vi "DataLogger_WriteData.vi"(8 "error in (no error)":errorcluster, 10 "New line":string, 11 "Data Logger in":refnum<class "Data Logger.lvclass">) -> (0 "error out":errorcluster, 3 "Data Logger out":refnum<class "Data Logger.lvclass">)   [LabVIEW 2015, in "Data Logger.lvclass"]
uses:
  Data Logger.lvclass
  Data Logger.lvclass/Data Logger.ctl
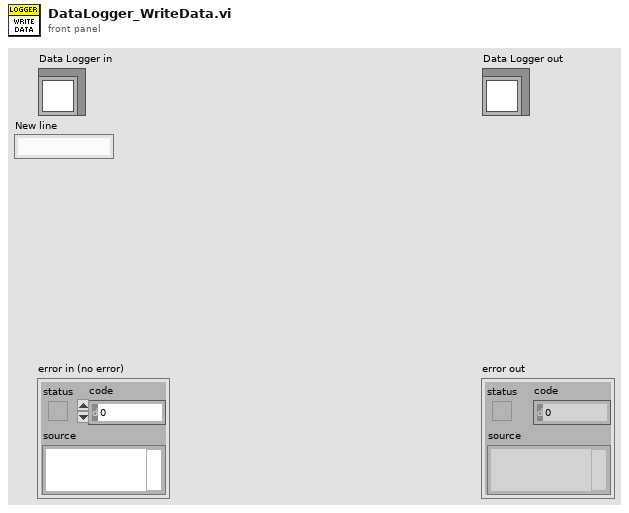
[diagram p1: front panel]
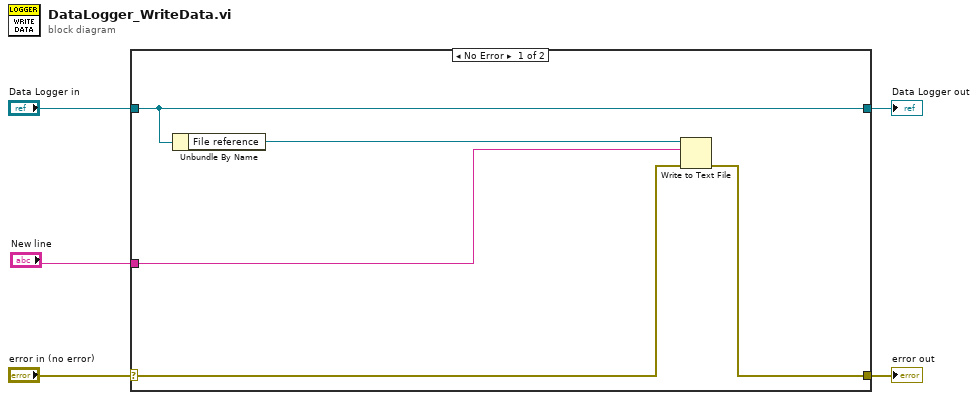
[diagram p0: block diagram]
diagram:
  n1 = case shown="No Error" "error in (no error)" {
    selector: "error in (no error)" -> [w8 w12]
    tunnel: [w7 w12] -> w4
    tunnel: [w10 w11] -> w2
    tunnel: "Data Logger in" -> [w10 w11]
    tunnel: "New line" -> [w6 _]
    frame No Error {
      n2 = Unbundle By Name(w10) -> ("File reference"=w9:refnum<file>)
      n3 = Write to Text File(file (use dialog)=w9, text=w6, error in=w8) -> (error out=w7:errorcluster)  [unwired: 1 in, 2 out]
    }
    frame Error {
    }
  }
  "error out" <- w4
  "Data Logger out" <- w2
